vi "Launch DeviceGUI.vi"(8 "error in (no error)":errorcluster, 11 "CS++DeviceActor in":refnum<class "CS++DeviceActor.lvclass">) -> (0 "error out":errorcluster, 3 "CS++DeviceActor out":refnum<class "CS++DeviceActor.lvclass">)   [LabVIEW 2012, in "CS++DeviceActor.lvlib" / "CS++DeviceActor.lvclass"]
doc: "Launch GUI for this device."
uses:
  CS++DeviceActor.lvclass
  CS++DeviceGUIActor/CS++DeviceGUIActor.lvclass
  CS++BaseActor/CS++BaseActor.lvclass/CS++BaseActor.ctl
  <vilib>/ActorFramework/Actor/Actor.lvclass/Actor.ctl
  <vilib>/ActorFramework/Message Enqueuer/Message Enqueuer.lvclass/Message Enqueuer.ctl
  CS++DeviceActor.lvclass/CS++DeviceActor.ctl
  CS++DeviceGUIActor/CS++DeviceGUIActor.lvclass/CS++DeviceGUIActor.ctl
  <vilib>/ActorFramework/Message Enqueuer/Init from Existing Queue.vi
  <vilib>/ActorFramework/Message Enqueuer/Message Enqueuer.lvclass
  <vilib>/ActorFramework/Actor/Actor.lvclass
  CS++BaseActor/CS++BaseActor.lvclass
  CS++BaseActor Messages/Open Actor Core FP Msg/Open Actor Core FP Msg.lvclass
panel:
  in  "Sub Panel":refnum<vi>
  in  "GUI Class Path":path
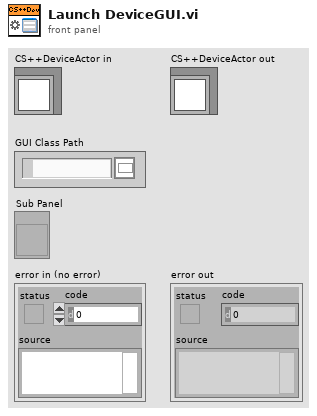
[diagram p1: front panel]
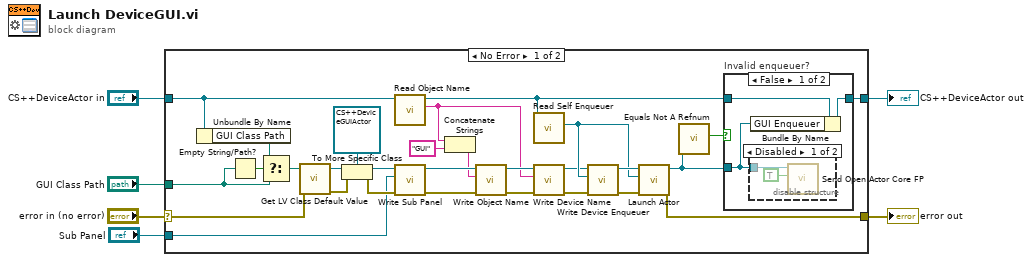
[diagram p0: block diagram]
diagram:
  n1 = case shown="No Error" "error in (no error)" {
    selector: "error in (no error)" -> [w31 w43]
    tunnel: [w26 w43] -> w5
    tunnel: [w27 w42] -> w3
    tunnel: "CS++DeviceActor in" -> [w15 w42]
    tunnel: "GUI Class Path" -> [w33 _]
    tunnel: "Sub Panel" -> [w21 _]
    frame No Error {
      n2 = Unbundle By Name(w15) -> ("GUI Class Path"=w34:path)
      n3 = Empty String/Path?(string/path=w33) -> (empty?=w35:bool)
      n4 = Select(t=w34, s=w35, f=w33) -> (s? t:f=w32:path)
      n5 = call <vilib>:"Get LV Class Default Value.vi"("error in (no error)"=w31, "class path"=w32) -> ("error out"=w29:errorcluster, "object"=w30:refnum<class>)  [unwired: 8 in]
      n6 = To More Specific Class(target class=refnum<class "CS++DeviceGUIActor.lvclass"> refnum ("CS++DeviceGUIActor.lvlib:CS++DeviceGUIActor.lvclass"), reference=w30, error in=w29) -> (specific class reference=w23:refnum<class "CS++DeviceGUIActor.lvclass">, error out=w22:errorcluster)
      n7 = call "Read Object Name.vi"("CS++BaseActor in"=w15) -> ("Object Name"=w9:string, "CS++BaseActor out"=w14:refnum<class "CS++DeviceActor.lvclass">)  [unwired: 8 in, 1 out]
      n8 = call "Write Sub Panel.vi"("error in (no error)"=w22, "Sub Panel"=w21, "CS++DeviceGUIActor in"=w23) -> ("error out"=w11:errorcluster, "CS++DeviceGUIActor out"=w13:refnum<class "CS++DeviceGUIActor.lvclass">)  [unwired: 7 in]
      n9 = Concatenate Strings(w9, "GUI" ("string")) -> (w7:string)
      n10 = call "Write Object Name.vi"("error in (no error)"=w11, "Object Name"=w7, "CS++BaseActor in"=w13) -> ("error out"=w10:errorcluster, "CS++BaseActor out"=w12:refnum<class "CS++DeviceGUIActor.lvclass">)  [unwired: 7 in]
      n11 = call <vilib>:"Read Self Enqueuer.vi"("Actor"=w14) -> ("Self Enqueuer"=w18:refnum<class "Message Enqueuer.lvclass">)  [unwired: 10 in]
      n12 = call "Write Device Name.vi"("error in (no error)"=w10, "Device Name"=w9, "CS++DeviceGUIActor in"=w12) -> ("error out"=w16:errorcluster, "CS++DeviceGUIActor out"=w17:refnum<class "CS++DeviceGUIActor.lvclass">)  [unwired: 7 in]
      n13 = call "Write Device Enqueuer.vi"("error in (no error)"=w16, "Device Enqueuer"=w18, "CS++DeviceGUIActor in"=w17) -> ("error out"=w19:errorcluster, "CS++DeviceGUIActor out"=w20:refnum<class "CS++DeviceGUIActor.lvclass">)  [unwired: 7 in]
      n14 = call <vilib>:"Launch Actor.vi"("error in (no error)"=w19, "Actor-to-Caller Enqueuer"=w18, "Actor"=w20) -> ("error out"=w26:errorcluster, "Caller-To-Actor Enqueuer"=w25:refnum<class "Message Enqueuer.lvclass">)  [unwired: 7 in]
      n15 = call <vilib>:"Equals Not A Refnum.vi"("Message Enqueuer"=w25) -> ("Not a refnum?"=w24:bool)  [unwired: 10 in]
      n16 = case "Invalid enqueuer?" shown="False" w24 {
        tunnel: w14 -> [w38 w41]
        tunnel: [w37 w41] -> w27
        tunnel: w25 -> [w36 _]
        frame False {
          n17 = disable-structure shown="Disabled" {
            disable-tunnel: w36 -> [w40 _]
            frame Disabled {
              n18 = call "Send Open Actor Core FP.vi"("Open FP (F)"=TRUE, "Message Enqueuer"=w40) -> ()  [unwired: 8 in, 2 out]
            }
            frame Enabled {
            }
          }
          n19 = Bundle By Name(cluster=w38, "GUI Enqueuer"=w36) -> (w37:refnum<class "CS++DeviceActor.lvclass">)
        }
        frame True {
        }
      }
    }
    frame Error {
    }
  }
  "error out" <- w5
  "CS++DeviceActor out" <- w3
